vi "顺序确定的日期查找算法.vi"() -> ()   [LabVIEW 2013]
panel:
  out "月段日":i32[](array[numeric])
  out "年段月":i32[](array[numeric])
  out "历史数据表格":i32(listbox)
  in  "数组":i32[][](array[numeric])=[[2015, 12, 27], [2015, 12, 16], [2015, 9, 16], [2015, 8, 14], [2014, 11, 7], [2014, 9, 3], [2014, 9, 25], [2014, 5, 16], [2013, 12, 7], [2012, 3, 3], [2010, 6, 5], [2010, 5, 9]]
  in  "日":u32
  in  "月":u32
  in  "年":u32
  in  "关闭":bool
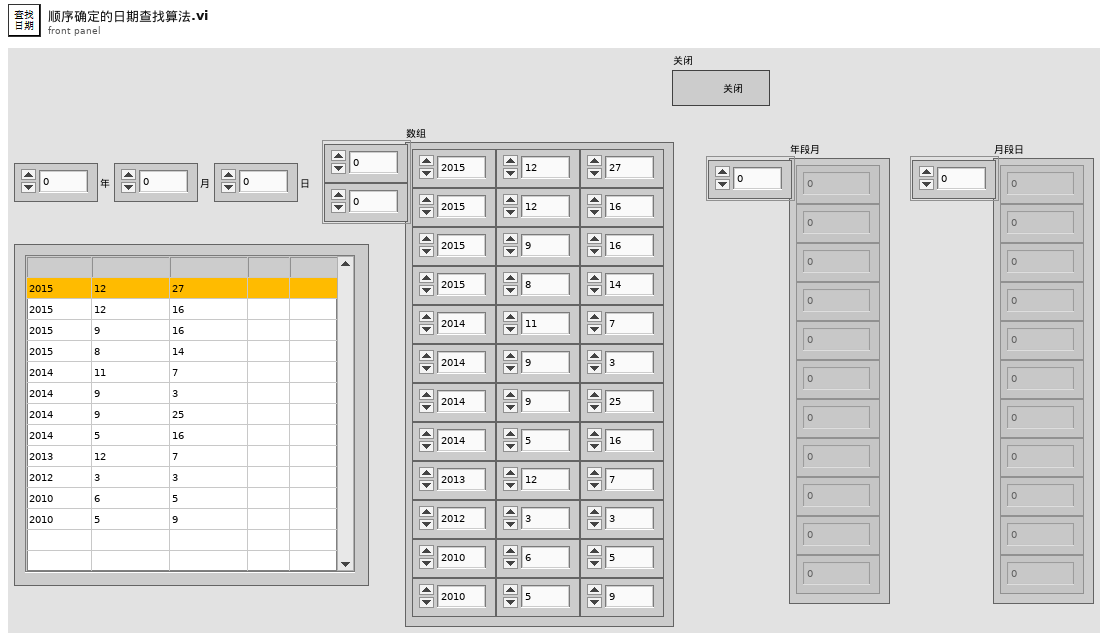
[diagram p1: front panel]
types:
  T1 = typedef "LVRowAndColumnUnsignedTypeDef.ctl" = cluster{"Row":u32, "Column":u32}
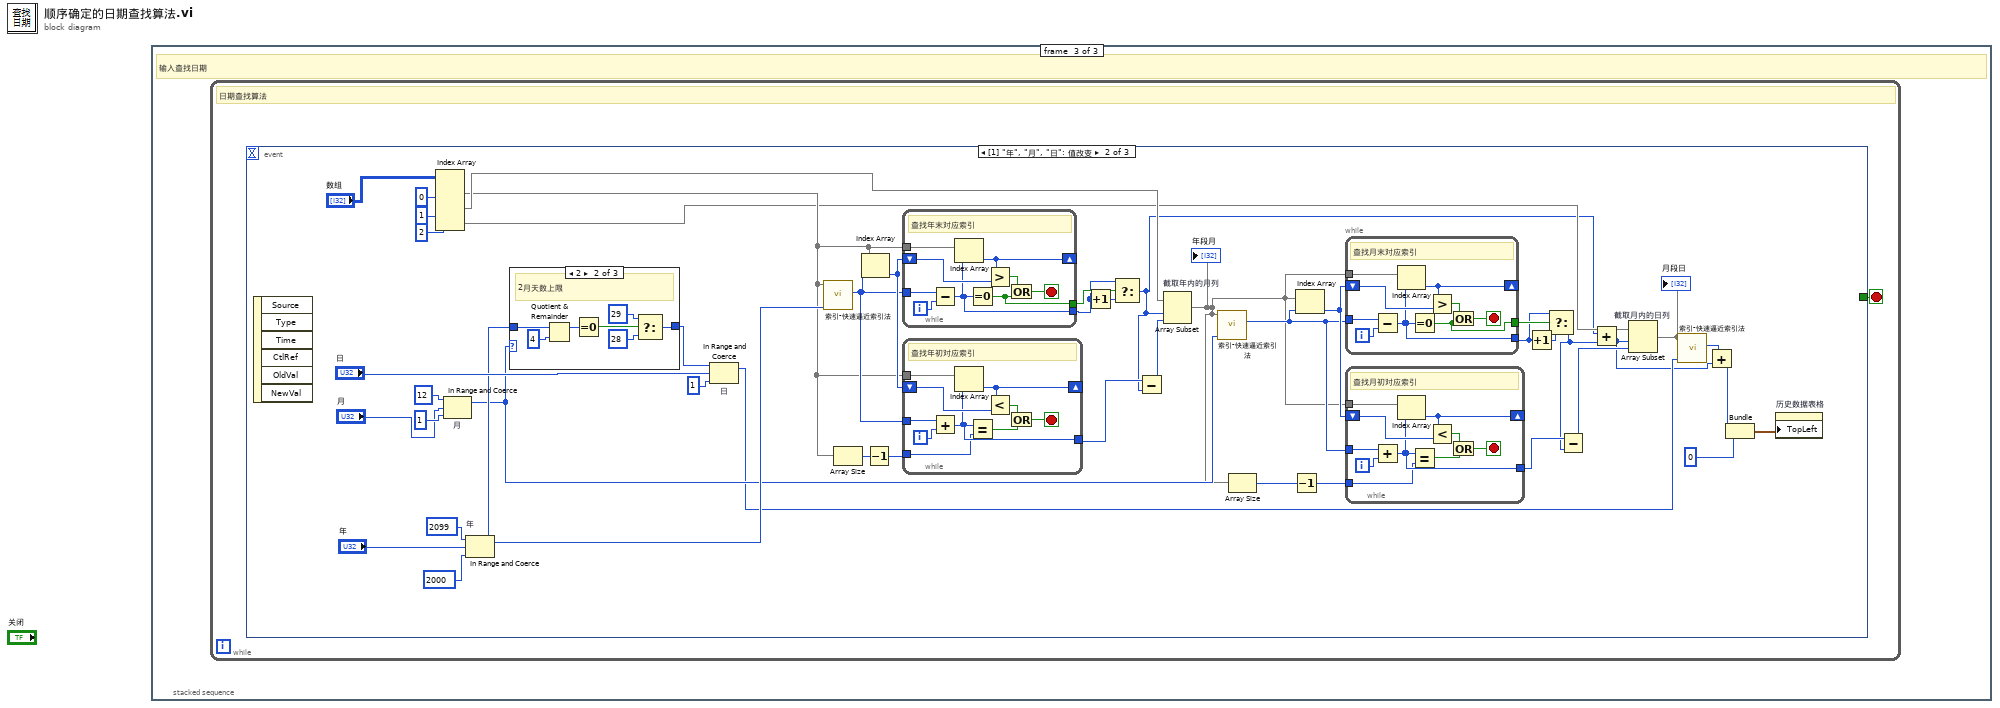
[diagram p0: block diagram]
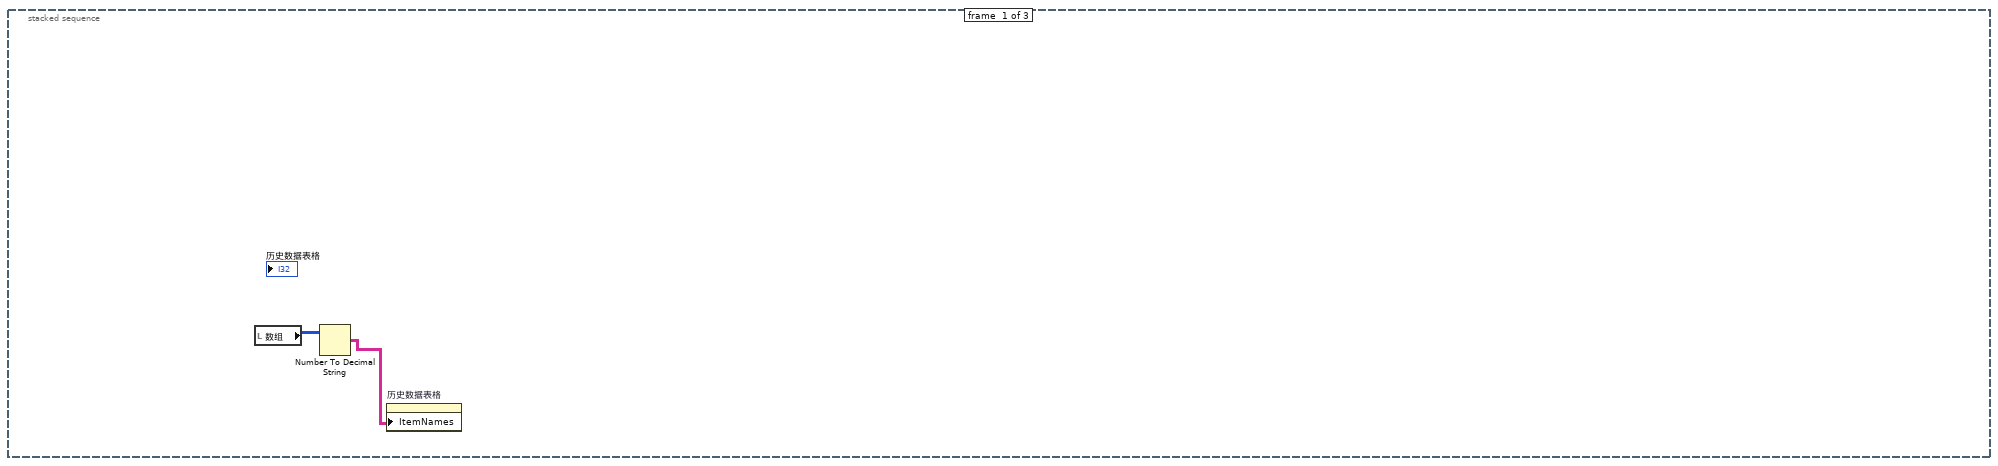
[diagram p2: hidden frame]
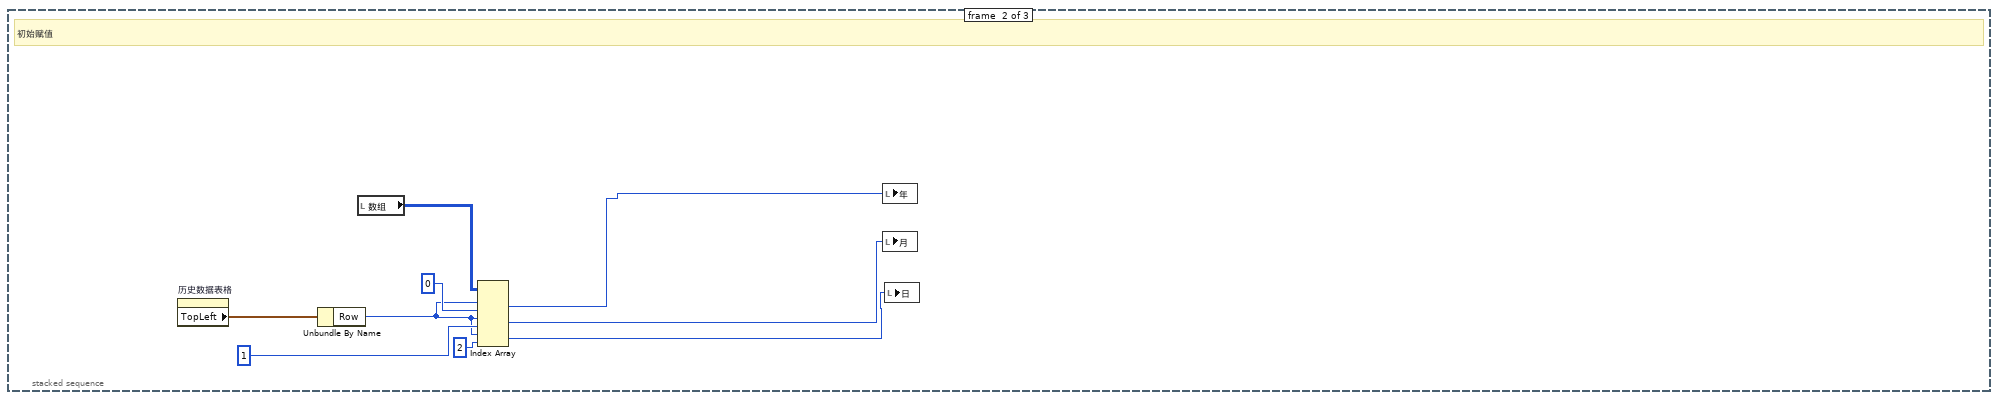
[diagram p3: hidden frame]
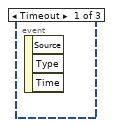
[diagram p4: hidden frame]
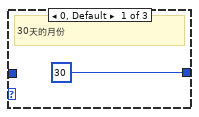
[diagram p5: hidden frame]
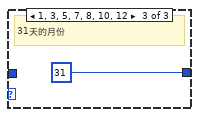
[diagram p6: hidden frame]
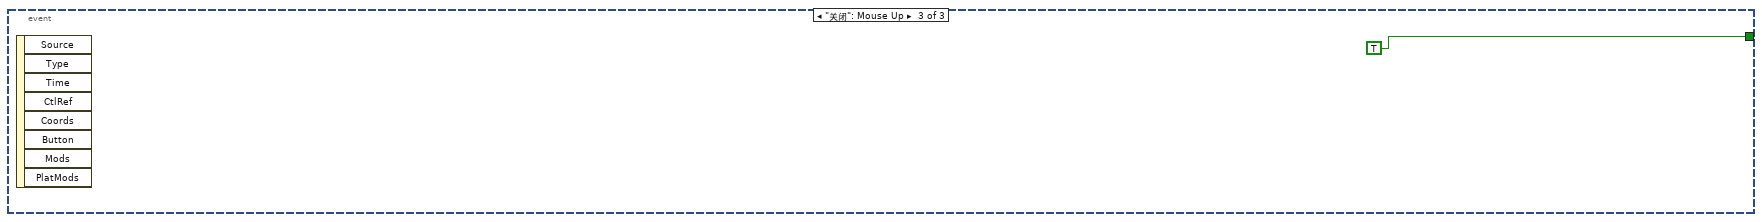
[diagram p7: hidden frame]
diagram:
  n1 = stacked-sequence {
    frame #0 {
      n2 = local read "数组"() -> (w1:i32[][])
      n3 = Number To Decimal String(number=w1) -> (decimal integer string=w2:string[][])  [unwired: 1 in]
      n4 = property on="历史数据表格" class="MCListbox (严格)"("ItemNames"=w2) -> ()  [unwired: 2 in, 2 out]
    }
    frame #1 {
      # "初始赋值"
      n5 = property on="历史数据表格" class="MCListbox (严格)"() -> ("TopLeft"=w8:T1)  [unwired: 2 in, 2 out]
      n6 = Unbundle By Name(w8) -> ("Row"=w7:u32)
      n7 = local read "数组"() -> (w6:i32[][])
      n8 = Index Array(array=w6, index (row) #1=w7, index (col) #1=0 ("禁用的索引 (列)"), index (row) #2=w7, index (col) #2=1 ("索引 (列)"), index (row) #3=w7, index (col) #3=2 ("索引 (列)")) -> (element #1=w5:i32, element #2=w4:i32, element #3=w3:i32)
      n9 = local write "年"(w5) -> ()
      n10 = local write "月"(w4) -> ()
      n11 = local write "日"(w3) -> ()
    }
    frame #2 {
      # "输入查找日期"
      n12 = while {
        stop <- w12 stop-if-true
        # "日期查找算法"
        n13 = event shown="[1] \"年\", \"月\", \"日\": 值改变" {
          selector: _ -> [_ _ _]
          dyn-events: _ -> [_ _ _]
          timeout: _ -> [_ _ _]
          tunnel: [_ _ TRUE] -> w12
          event Timeout {
            n14 = event-data() -> ()  [unwired: 1 in, 3 out]
          }
          event "年", "月", "日": Value Change {
            n15 = event-data() -> ()  [unwired: 1 in, 6 out]
            n16 = Index Array(array="数组", index (col) #1=0 ("禁用的索引 (列)"), index (col) #2=1 ("索引 (列)"), index (col) #3=2 ("索引 (列)")) -> (element #1=w33:i32[], element #2=w39:i32[], element #3=w29:i32[])  [unwired: 3 in]
            n17 = In Range and Coerce "月"(upper limit=u32 12 ("上限"), x="月", lower limit=u32 1 ("上限")) -> (coerced(x)=w38:u32)  [unwired: 1 out]
            n18 = In Range and Coerce "年"(upper limit=u32 2099 ("上限"), x="年", lower limit=u32 2000 ("下限")) -> (coerced(x)=w46:u32)  [unwired: 1 out]
            n19 = case shown="2" w38 {
              tunnel: [u32 30 ("上限") w101 u32 31 ("上限")] -> w53
              tunnel: w46 -> [_ w104 _]
              frame 0, Default {
                # "30天的月份"
              }
              frame 2 {
                # "2月天数上限"
                n20 = Quotient & Remainder(x=w104, y=u32 4) -> (x-y*floor(x/y)=w102:u32)  [unwired: 1 out]
                n21 = Equal To 0?(x=w102) -> (x = 0?=w100:bool)
                n22 = Select(t=u32 29, s=w100, f=u32 28 ("t")) -> (s? t:f=w101:u32)
              }
              frame 1, 3, 5, 7, 8, 10, 12 {
                # "31天的月份"
              }
            }
            n23 = In Range and Coerce "日"(upper limit=w53, x="日", lower limit=u32 1 ("上限")) -> (coerced(x)=w27:u32)  [unwired: 1 out]
            n24 = call "索引-快速逼近索引法.vi"("数值"=w46, "数组"=w33) -> ("最近索引"=w44:i32)  [unwired: 9 in]
            n25 = Array Size(array=w33) -> (size(s)=w43:i32)
            n26 = Index Array(array=w33, index=w44) -> (element=w45:i32)
            n27 = Decrement(x=w43) -> (x-1=w42:i32)
            n28 = while {
              tunnel: w44 -> [w96]
              tunnel: w33 -> [w94]
              shift-right: [w93] -> _
              shift-left: w45 -> [w92]
              tunnel: [w89] -> w21
              tunnel: [w88] -> w22
              i -> [w95]
              stop <- w90 stop-if-true
              # "查找年末对应索引"
              n29 = Subtract(x=w96, y=w95) -> (x-y=w89:i32)
              n30 = Index Array(array=w94, index=w89) -> (element=w93:i32)
              n31 = Equal To 0?(x=w89) -> (x = 0?=w88:bool)
              n32 = Greater?(x=w93, y=w92) -> (0:w91:bool)
              n33 = Or(x=w91, y=w88) -> (x .or. y?=w90:bool)
            }
            n34 = while {
              tunnel: w44 -> [w87]
              tunnel: w33 -> [w85]
              shift-right: [w84] -> _
              shift-left: w45 -> [w83]
              tunnel: [w79] -> w41
              tunnel: w42 -> [w78]
              i -> [w86]
              stop <- w80 stop-if-true
              # "查找年初对应索引"
              n35 = Add(x=w87, y=w86) -> (x+y=w79:i32)
              n36 = Index Array(array=w85, index=w79) -> (element=w84:i32)
              n37 = Equal?(x=w79, y=w78) -> (x = y?=w81:bool)
              n38 = Less?(x=w84, y=w83) -> (x < y?=w82:bool)
              n39 = Or(x=w82, y=w81) -> (x .or. y?=w80:bool)
            }
            n40 = Increment(x=w21) -> (x+1=w20:i32)
            n41 = Select(t=w21, s=w22, f=w20) -> (s? t:f=w15:i32)
            n42 = Subtract(x=w41, y=w15) -> (x-y=w40:i32)
            n43 = Array Subset "截取年内的月列"(array=w39, index=w15, length=w40) -> (w32:i32[])
            "年段月" <- w32
            n44 = call "索引-快速逼近索引法.vi"("数值"=w38, "数组"=w32) -> ("最近索引"=w35:i32)  [unwired: 9 in]
            n45 = Array Size(array=w32) -> (size(s)=w37:i32)
            n46 = Decrement(x=w37) -> (x-1=w34:i32)
            n47 = Index Array(array=w32, index=w35) -> (element=w36:i32)
            n48 = while {
              tunnel: w35 -> [w77]
              tunnel: w32 -> [w75]
              shift-right: [w74] -> _
              shift-left: w36 -> [w73]
              tunnel: [w70] -> w17
              tunnel: [w69] -> w19
              i -> [w76]
              stop <- w71 stop-if-true
              # "查找月末对应索引"
              n49 = Subtract(x=w77, y=w76) -> (x-y=w70:i32)
              n50 = Index Array(array=w75, index=w70) -> (element=w74:i32)
              n51 = Equal To 0?(x=w70) -> (x = 0?=w69:bool)
              n52 = Greater?(x=w74, y=w73) -> (0:w72:bool)
              n53 = Or(x=w72, y=w69) -> (x .or. y?=w71:bool)
            }
            n54 = while {
              tunnel: w35 -> [w68]
              tunnel: w32 -> [w66]
              shift-right: [w65] -> _
              shift-left: w36 -> [w64]
              tunnel: [w60] -> w31
              tunnel: w34 -> [w59]
              i -> [w67]
              stop <- w61 stop-if-true
              # "查找月初对应索引"
              n55 = Add(x=w68, y=w67) -> (x+y=w60:i32)
              n56 = Index Array(array=w66, index=w60) -> (element=w65:i32)
              n57 = Equal?(x=w60, y=w59) -> (x = y?=w62:bool)
              n58 = Less?(x=w65, y=w64) -> (x < y?=w63:bool)
              n59 = Or(x=w63, y=w62) -> (x .or. y?=w61:bool)
            }
            n60 = Increment(x=w17) -> (x+1=w18:i32)
            n61 = Select(t=w17, s=w19, f=w18) -> (s? t:f=w16:i32)
            n62 = Subtract(x=w31, y=w16) -> (x-y=w30:i32)
            n63 = Add(x=w15, y=w16) -> (x+y=w13:i32)
            n64 = Array Subset "截取月内的日列"(array=w29, index=w13, length=w30) -> (w28:i32[])
            "月段日" <- w28
            n65 = call "索引-快速逼近索引法.vi"("数值"=w27, "数组"=w28) -> ("最近索引"=w26:i32)  [unwired: 9 in]
            n66 = Add(x=w26, y=w13) -> (x+y=w14:i32)
            n67 = Bundle(w14, "最近索引"=0) -> (w23:cluster{i32, "最近索引":i32})  [unwired: 1 in]
            n68 = property on="历史数据表格" class="MCListbox (严格)"("TopLeft"=w23) -> ()  [unwired: 2 in, 2 out]
          }
          event "关闭": Mouse Up {
            n69 = event-data() -> ()  [unwired: 1 in, 8 out]
          }
        }
      }
    }
  }
